vi "fixedPoint.vi"() -> ()   [LabVIEW 2018]
uses:
  <vilib>/Platform/TimedLoop/XDataNode/timing_clust.ctl
  <vilib>/Platform/TimedLoop/XDataNode/nitl_modes.ctl
  <vilib>/Platform/TimedLoop/XDataNode/wakeup.ctl
  <vilib>/rvi/Emulation/niFpgaSctlEmulationGetInTimedLoop.vi
  <vilib>/rvi/Emulation/niFpgaEmulationReportErrorSimple.vi
  <vilib>/rvi/Emulation/niFpgaGetClockAttributes.vi
  <vilib>/rvi/Emulation/niFpgaCriticalErrorInLSC.vi
  lib/Cast-EPICS/cast u-64-64 to u64.vi
  lib/Cast-EPICS/cast u-64-0 to u64.vi
  lib/Cast-EPICS/cast u-64-32 to u64.vi
  lib/Cast-EPICS/cast s-64-0 to u64.vi
  lib/Cast-EPICS/cast s-64-64 to u64.vi
  lib/Cast-EPICS/cast s-64-32 to u64.vi
  <vilib>/Platform/TimedLoop/XDataNode/XDataNode.xnode
  <vilib>/Platform/TimedLoop/XDataNode/XDNodeRunTimeDep.lvlib
  lib/Cast-EPICS/fixedpoint-cast.lvlib
panel:
  out "aifxp 6":u64
  in  "fixedpoint_i 6":fxp<+/-,64,32> format="%#_20g"
  out "aifxp 5":u64
  in  "fixedpoint_i 5":fxp<+/-,64,64> format="%.20f"
  out "aifxp 4":u64
  in  "fixedpoint_i 4":fxp<+/-,64,0> format="%#_20g"
  out "aifxp 3":u64
  in  "fixedpoint_i 3":fxp<+,64,32> format="%#_20g"
  out "aifxp 2":u64
  in  "fixedpoint_i 2":fxp<+,64,0> format="%#_20g"
  out "aifxp":u64
  in  "fixedpoint_i":fxp<+,64,64> format="%.20f"
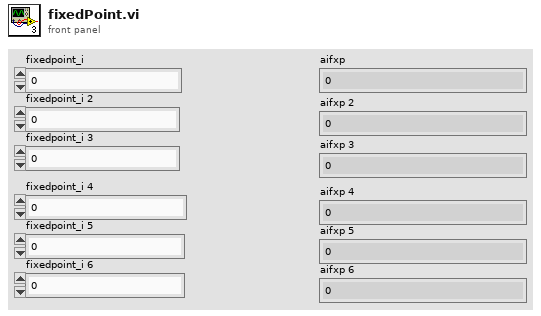
[diagram p1: front panel]
types:
  T1 = typedef "XDNodeRunTimeDep.lvlib/timing_clust.ctl" = cluster{"Expected End [f-1]":u64, "Actual End [f-1]":u64, "Finished Late? [f-1]":bool, "Expected End [i-1]":u64, "Actual End [i-1]":u64, "Finished Late? [i-1]":bool, "Expected Start [i]":u64, "Actual Start [i]":u64, "Expected Start [f]":u64, "Actual Start [f]":u64, "Source Name":string, "Structure Name":string, "Period":i64, "Deadline":i64, "Offset":i64, "Start":i64, "Priority":i32, "Timeout":i32, "Mode":T2, "Wakeup Reason":T3, "Error":errorcluster, "Source Type":string, "Secondary Source Type":string, "Global End Time":u64, "Global Start Time":u64, "Frame Duration":u64, "Iteration Duration":u64, "Assigned CPU":i32, "I/O Scan Engine Mode":u32}
  T2 = typedef "XDNodeRunTimeDep.lvlib/nitl_modes.ctl" = enum32{"No Change", "Process missed periods, maintain original phase", "Discard missed periods, maintain original phase", "Process missed periods, ignore original phase", "Discard missed periods, ignore original phase"}
  T3 = typedef "XDNodeRunTimeDep.lvlib/wakeup.ctl" = enum32{"Normal", "Aborted", "Asynchronous wakeup", "Timing source error", "Timed loop error", "Timeout"}
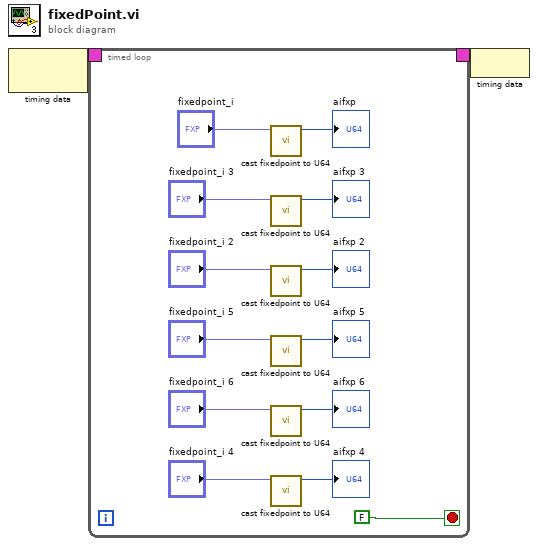
[diagram p0: block diagram]
diagram:
  n1 = node-c288() -> (w2:T1)  [unwired: 1 in]
  n2 = timed-loop {
    timing: w2 -> [_]
    timing-out: [_] -> w1
    stop <- FALSE stop-if-true
    n3 = call-poly "cast fixedpoint to U64.vi"("fixedpoint_i"="fixedpoint_i") -> ("aifxp"=→"aifxp":u64)  [unwired: 10 in]
    n4 = call-poly "cast fixedpoint to U64.vi"("fixedpoint_i"="fixedpoint_i 3") -> ("aifxp"=→"aifxp 3":u64)  [unwired: 10 in]
    n5 = call-poly "cast fixedpoint to U64.vi"("fixedpoint_i"="fixedpoint_i 2") -> ("aifxp"=→"aifxp 2":u64)  [unwired: 10 in]
    n6 = call-poly "cast fixedpoint to U64.vi"("fixedpoint_i"="fixedpoint_i 5") -> ("aifxp"=→"aifxp 5":u64)  [unwired: 10 in]
    n7 = call-poly "cast fixedpoint to U64.vi"("fixedpoint_i"="fixedpoint_i 6") -> ("aifxp"=→"aifxp 6":u64)  [unwired: 10 in]
    n8 = call-poly "cast fixedpoint to U64.vi"("fixedpoint_i"="fixedpoint_i 4") -> ("aifxp"=→"aifxp 4":u64)  [unwired: 10 in]
  }
  n9 = node-c288(w1) -> ()
